vi "get_width_from_zero.vi"(8 "dt":dbl, 10 "minus-plus crossing?":bool[](array[boolean]), 11 "plus-minus crossing?":bool[](array[boolean])) -> (0 "variance of width":dbl format="%0.2f", 1 "sd of width":dbl format="%0.2f", 2 "mean of width":dbl format="%0.2f", 3 "width":dbl[](array[numeric]), 4 "width graph":cluster{i32[], dbl[]}(graph))   [LabVIEW 2020]
uses:
  <vilib>/Analysis/NI_AALBase.lvlib
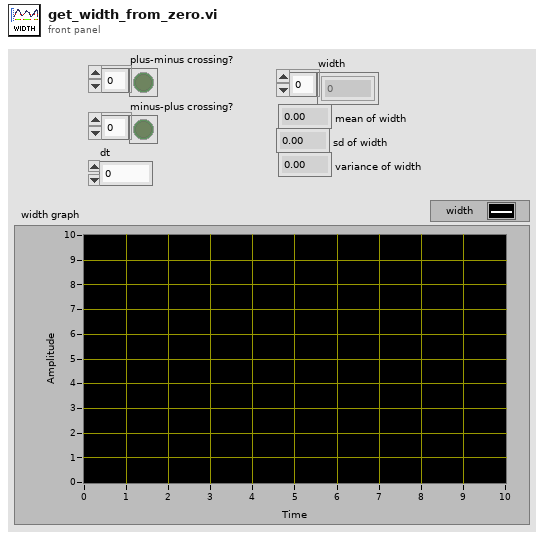
[diagram p1: front panel]
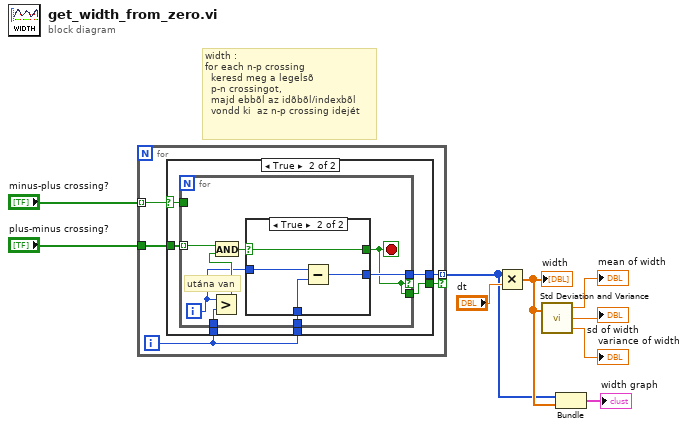
[diagram p0: block diagram]
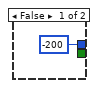
[diagram p2: hidden frame]
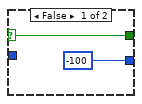
[diagram p3: hidden frame]
diagram:
  # "width :\nfor each n-p crossing\n  keresd meg a legelsõ\n  p-n crossingot,\n  majd ebbõl az idõbõl/indexbõl\n  vondd ki  az n-p crossing idejét"
  n1 = for {
    tunnel: "minus-plus crossing?" -> [w13] mode=indexing
    tunnel: "plus-minus crossing?" -> [w14]
    tunnel: [w11] -> w1 mode=indexing if=w10
    i -> [w12]
    n2 = case shown="True" w13 {
      selector: w13 -> [_ w20]
      tunnel: w14 -> [_ w21]
      tunnel: w12 -> [_ w19]
      tunnel: w12 -> [_ w18]
      tunnel: [-200 w17] -> w11
      tunnel: [_ w16] -> w10
      frame False {
      }
      frame True {
        n3 = for {
          tunnel: w21 -> [w28] mode=indexing
          tunnel: w20 -> [_]
          tunnel: w19 -> [w29]
          tunnel: w18 -> [w25]
          tunnel: [w23] -> w17 if=w22
          tunnel: [w22] -> w16
          i -> [w24]
          stop <- w22 stop-if-true
          # "utána van"
          n4 = Greater?(x=w24, y=w29) -> (0:w27:bool)
          n5 = And(x=w28, y=w27) -> (x .and. y?=w26:bool)
          n6 = case shown="True" w26 {
            selector: w26 -> [w31 w32]
            tunnel: w25 -> [_ w34]
            tunnel: w24 -> [_ w35]
            tunnel: [-100 w33] -> w23
            tunnel: [w31 w32] -> w22
            frame False {
            }
            frame True {
              n7 = Subtract(x=w35, y=w34) -> (x-y=w33:i32)
            }
          }
        }
      }
    }
  }
  n8 = Multiply(x=w1, y="dt") -> (x*y=w2:dbl[])
  "width" <- w2
  n9 = call <vilib>:"Std Deviation and Variance.vi"("X"=w2) -> ("mean"=→"mean of width":dbl, "standard deviation"=→"sd of width":dbl, "variance"=→"variance of width":dbl)  [unwired: 1 in]
  n10 = Bundle(w1, w2) -> (→"width graph":cluster{i32[], dbl[]})  [unwired: 1 in]
